vi "PowerSupply.vi"(7 "LWSR":refnum<class "Web Request.lvclass">, 11 "val":u8) -> ()   [LabVIEW 2014]
uses:
  <vilib>/wsapi/Web Request.lvclass
  Controller/Messages/Power Supply/PowerSupply MSG.lvclass
  Controller/Controller.lvclass
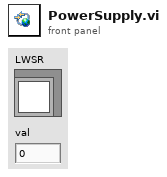
[diagram p1: front panel]
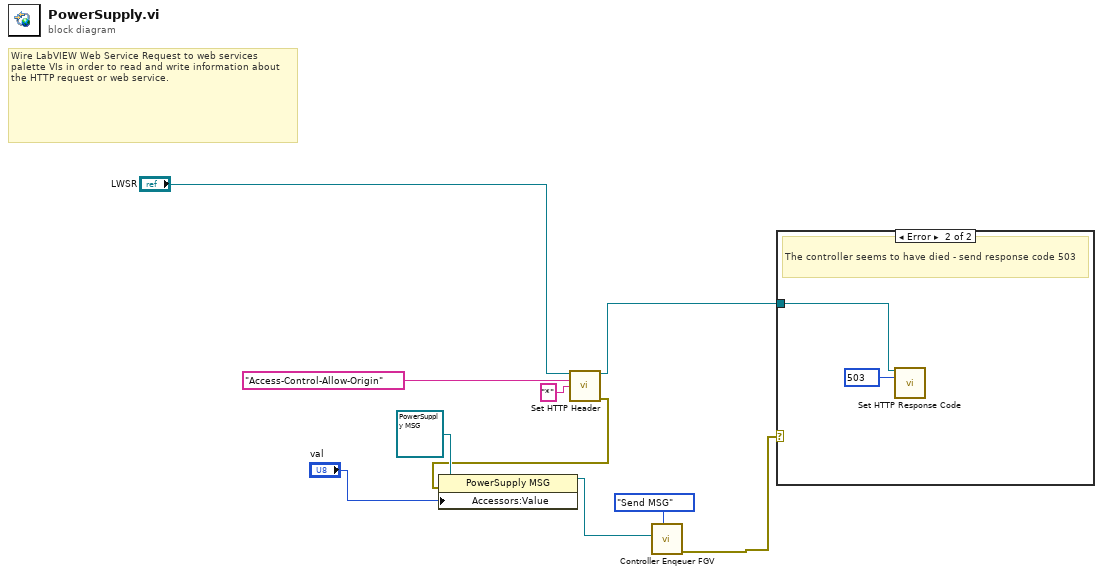
[diagram p0: block diagram]
diagram:
  # "Wire LabVIEW Web Service Request to web services palette VIs in order to read and write information about the HTTP request or web service."
  n1 = call <vilib>:"Set HTTP Header.vi"("LabVIEW Web Service Request"="LWSR", "header"="Access-Control-Allow-Origin", "header value"="*") -> ("LabVIEW Web Service Request out"=w1:refnum<class "Web Request.lvclass">, "error out"=w5:errorcluster)  [unwired: 11 in]
  n2 = property class="PowerSupply MSG"(reference=refnum<class "PowerSupply MSG.lvclass"> refnum ("Controller.lvlib:PowerSupply MSG"), error in=w5, "Accessors:Value"="val") -> (reference out=w4:refnum<class "PowerSupply MSG.lvclass">)  [unwired: 1 out]
  n3 = call "Controller Enqeuer FGV.vi"("State"=enum16{"Store", "Send MSG"}."Send MSG", "MSG"=w4) -> ("error out"=w2:errorcluster)  [unwired: 9 in]
  n4 = case shown="Error" w2 {
    tunnel: w1 -> [_ w11]
    frame No Error {
    }
    frame Error {
      w12 = 503 items=["100"=100, "101"=101, "200"=200, "201"=201, "202"=202, "203"=203, "204"=204, "205"=205, "206"=206, "300"=300, "301"=301, "302"=302, "303"=303, "304"=304, "305"=305, "306"=306, "307"=307, "400"=400, "401"=401, "402"=402, "403"=403, "404"=404, "405"=405, "406"=406, "407"=407, "408"=408, "409"=409, "410"=410, "411"=411, "412"=412, "413"=413, "414"=414, "415"=415, "416"=416, "417"=417, "500"=500, "501"=501, "502"=502, "503"=503, "504"=504, "505"=505] ("response code (200)")
      # "The controller seems to have died - send response code 503"
      n5 = call <vilib>:"Set HTTP Response Code.vi"("LabVIEW Web Service Request"=w11, "response code (200)"=w12) -> ()  [unwired: 12 in, 2 out]
    }
  }
